vi "Double FFT Mesurament (Max Bin detection & CLK trick) test.vi"   [LabVIEW 2014]
uses:
  <vilib>/Platform/TimedLoop/XDataNode/timing_clust.ctl
  <vilib>/Platform/TimedLoop/XDataNode/nitl_modes.ctl
  <vilib>/Platform/TimedLoop/XDataNode/wakeup.ctl
  <vilib>/rvi/Analysis/measure/FFT/simModelSupport/niFPGA FFT Streaming Sim Properties.ctl
  <vilib>/rvi/Analysis/measure/FFT/simModelSupport/niFPGA FFT Sim Stream Group Properties.ctl
  <vilib>/rvi/Analysis/measure/FFT/simModelSupport/niFPGA FFT Sim Types.ctl
  <vilib>/rvi/Analysis/measure/FFT/simModelSupport/niFpgaFFTSimArithmeticProperties.ctl
  <vilib>/rvi/Analysis/measure/FFT/simModelSupport/niFpgaFFTSimDfxp.ctl
  <vilib>/fxp/LVFixedPointQuantizationPolicyTypeDef.ctl
  <vilib>/rvi/Analysis/measure/FFT/XNode/niFpgaFFTButterflyDelays.ctl
  <vilib>/rvi/Emulation/niFpgaSctlEmulationGetInTimedLoop.vi
  <vilib>/rvi/Emulation/niFpgaEmulationReportErrorSimple.vi
  <vilib>/rvi/Emulation/niFpgaGetClockAttributes.vi
  <vilib>/rvi/Emulation/niFpgaCriticalErrorInLSC.vi
  <vilib>/rvi/eio/common/nirviEmuTemplateMethod_errors.vi
  <vilib>/rvi/Emulation/niFpgaEmulationIsFPGAContextNoSignature.vi
  <vilib>/rvi/errors/niFpgaSetErrorForExecOnDevCompSimple.vi
  <vilib>/rvi/eio/common/nirviEmuReportErrorAndStop.vi
  <vilib>/rvi/DataTransferAndStorage/Container/Common/niFpgaContainerGetUniqueNameForEmu.vi
  <vilib>/rvi/FIFO/Fifo_Resource/nirvififoEmulationSetSize.vi
  <vilib>/rvi/FIFO/Fifo_Resource/nirviFifoEmulationQueueMgr.vi
  <instcachedir>/0/nirviFifoEmulationQueueMgr_E5CAEC123FF24DC58D834DCA3CDAA9B5.lvgen/nirviFifoEmulationQueueMgr_E5CAEC123FF24DC58D834DCA3CDAA9B5_005.vi
  <vilib>/Utility/error.llb/Clear Errors.vi
  <vilib>/rvi/FIFO/Fifo_Resource/nirvififoEmulationCreateLock.vi
  <vilib>/rvi/Emulation/niFpgaProcessEmulError.vi
  <vilib>/rvi/FIFO/Fifo_Resource/nirvififoEmulationObtainLock.vi
  <vilib>/rvi/FIFO/Fifo_Resource/nirvififoEmulationReleaseLock.vi
  <vilib>/rvi/occurrence/nirviWaitOnOccurrenceBase.vi
  <vilib>/rvi/errors/nirviReportUnexpectedCaseInternalError.vi
  <vilib>/rvi/errors/nirviReportUnexpectedCaseInternalError (U32).vi
  <vilib>/rvi/Memory/Memory_Emulation/niFpgaMemoryEmulationCacheClearOnFirstRun.vi
  <vilib>/rvi/Memory/Memory_Emulation/nirvimemoryEmulationManagerCache_MakeExclusive.vi
  <vilib>/rvi/Memory/Memory_Emulation/niFpgaMemoryEmulationValidateCache.vi
  <vilib>/rvi/Memory/Memory_Emulation/nirvimemoryEmulationManagerCache_InsertValue.vi
  <vilib>/rvi/Memory/Memory_Emulation/nirvimemoryEmulationManagerCache_ReleaseExclusive.vi
  <vilib>/rvi/Memory/Memory_Emulation/nirvimemoryEmulationManagerCache_GetValue.vi
  <vilib>/rvi/Memory/Memory_Emulation/nirvimemoryEmulationManagerCache_SetValue.vi
  <instcachedir>/0/nirviFifoEmulationQueueMgr_E5CAEC123FF24DC58D834DCA3CDAA9B5.lvgen/nirviFifoEmulationQueueMgr_E5CAEC123FF24DC58D834DCA3CDAA9B5_004.vi
  <vilib>/rvi/FIFO/Fifo_Resource/nirvififoEmulationDetermineInputValidOut.vi
  <vilib>/rvi/Memory/Memory_Emulation/nirvimemoryFastEmulation.vi
  <vilib>/rvi/Memory/Memory_Emulation/nirvimemoryEmulation.vi
  <vilib>/rvi/Analysis/measure/FFT/simModelSupport/niFpgaFFTSimModelStreamingCore.vi
  <vilib>/Platform/TimedLoop/XDataNode/XDataNode.xnode
  <vilib>/eio/EIOMethodNode/EIOMethodNode.xnode
  <vilib>/rvi/DataTransferAndStorage/Container/XNode/niFpgaContainer.xnode
  <vilib>/rvi/FIFO/Fifo_Resource/nirvififoEmulationRead.vi
  <vilib>/rvi/DataTransferAndStorage/Register/Emulation/niFpgaRegisterEmulation.vi
  <vilib>/rvi/FIFO/Fifo_Resource/nirvififoEmulationWrite.vi
  <vilib>/rvi/FIFO/Fifo_Resource/nirvififoEmulationGetNumberOfElementsToWrite.vi
  <vilib>/rvi/Analysis/measure/FFT/XNode/niFpgaFFT.xnode
  <vilib>/Platform/TimedLoop/XDataNode/XDNodeRunTimeDep.lvlib
types:
  T1 = typedef "XDNodeRunTimeDep.lvlib/timing_clust.ctl" = cluster{"Expected End [f-1]":u64, "Actual End [f-1]":u64, "Finished Late? [f-1]":bool, "Expected End [i-1]":u64, "Actual End [i-1]":u64, "Finished Late? [i-1]":bool, "Expected Start [i]":u64, "Actual Start [i]":u64, "Expected Start [f]":u64, "Actual Start [f]":u64, "Source Name":string, "Structure Name":string, "Period":i64, "Deadline":i64, "Offset":i64, "Start":i64, "Priority":i32, "Timeout":i32, "Mode":T2, "Wakeup Reason":T3, "Error":errorcluster, "Source Type":string, "Secondary Source Type":string, "Global End Time":u64, "Global Start Time":u64, "Frame Duration":u64, "Iteration Duration":u64, "Assigned CPU":i32, "I/O Scan Engine Mode":u32}
  T2 = typedef "XDNodeRunTimeDep.lvlib/nitl_modes.ctl" = enum32{"No Change", "Process missed periods, maintain original phase", "Discard missed periods, maintain original phase", "Process missed periods, ignore original phase", "Discard missed periods, ignore original phase"}
  T3 = typedef "XDNodeRunTimeDep.lvlib/wakeup.ctl" = enum32{"Normal", "Aborted", "Asynchronous wakeup", "Timing source error", "Timed loop error", "Timeout"}
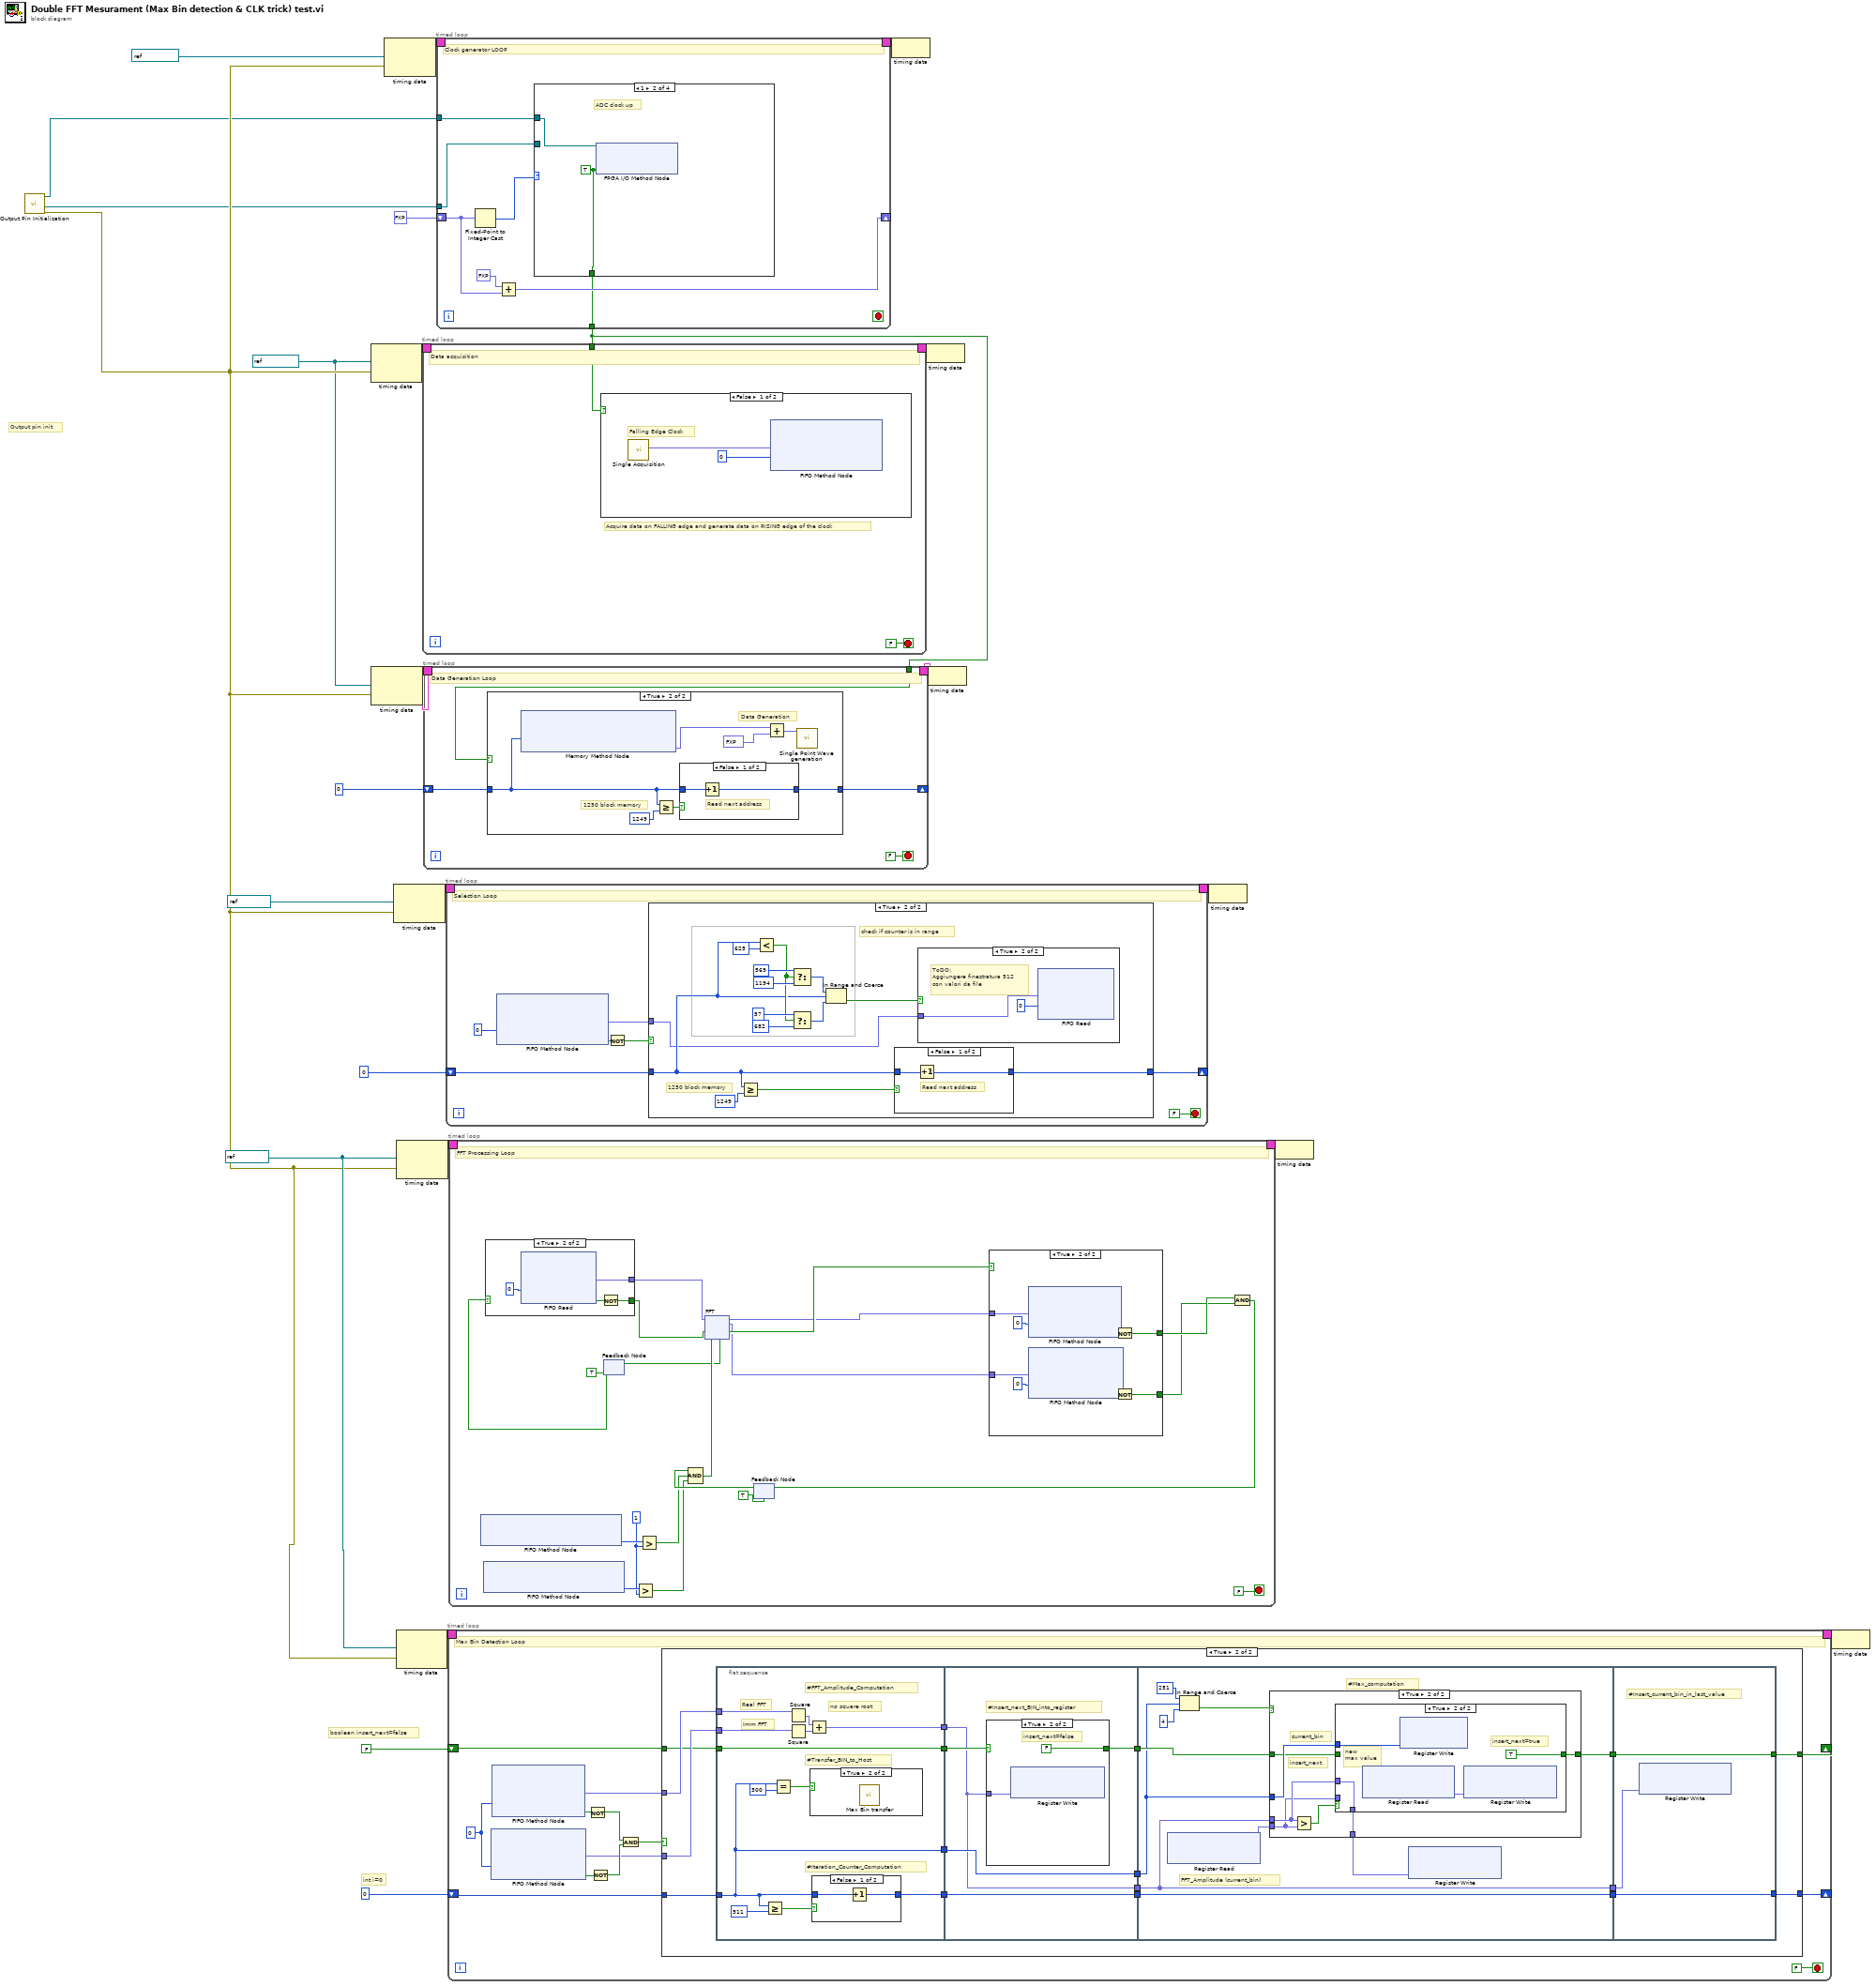
[diagram p0: block diagram]
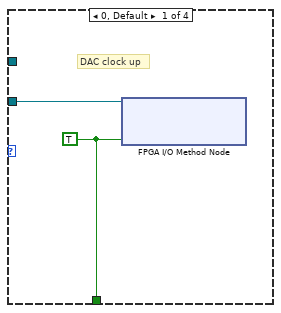
[diagram p2: hidden frame]
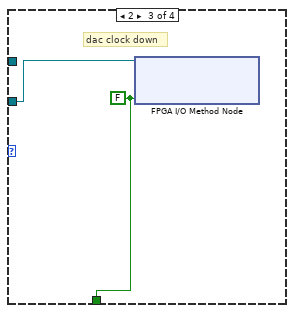
[diagram p3: hidden frame]
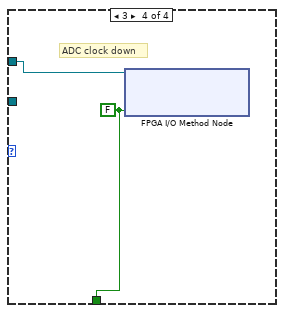
[diagram p4: hidden frame]
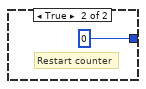
[diagram p7: hidden frame]
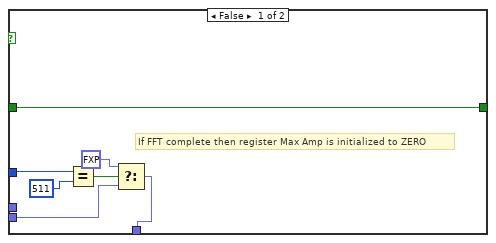
[diagram p9: hidden frame]
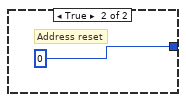
[diagram p13: hidden frame]
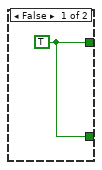
[diagram p14: hidden frame]
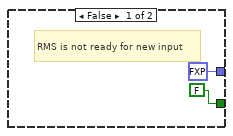
[diagram p15: hidden frame]
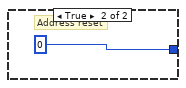
[diagram p17: hidden frame]
diagram:
  w11 = refnum<k21> "50MHz" ("Source Name")
  w2 = refnum<k21> "100MHz" ("Source Name")
  # "int i=0"
  # "boolean insert_next=false"
  # "Output pin init"
  n1 = call "Output Pin Initialization.vi"() -> ("error out"=w7:errorcluster, "I/O Out Clock DAC (pin16)"=w5:refnum<k21>, "I/O Out Clock ADC (pin17)"=w4:refnum<k21>)  [unwired: 8 in]
  n2 = node-c288(w2, w7) -> (w25:T1)
  n3 = node-c288(w2, w7) -> (w23:T1)
  n4 = node-c288(refnum<k21> "200MHz" ("Source Name"), w7) -> (w10:T1)
  n5 = node-c288(refnum<k21> "50MHz" ("Source Name"), w7) -> (w19:T1)
  n6 = node-c288(w11, w7) -> (w13:T1)
  n7 = node-c288(w11, w7) -> (w21:T1)
  n8 = timed-loop {
    timing: w10 -> [_]
    timing-out: [_] -> w9
    shift-right: [w29] -> _
    shift-left: fxp<+,2,2> 0.0 -> [w31]
    tunnel: w5 -> [w28]
    tunnel: [w27] -> w3
    tunnel: w4 -> [w26]
    stop <- _ stop-if-true
    # "Clock generator LOOP"
    n9 = Fixed-Point to Integer Cast(1:w31) -> (0:w32:u8)
    n10 = Add(x=fxp<+,2,2> 1.0, y=w31) -> (x+y=w29:fxp<+,2,2>)
    n11 = case shown="1" w32 {
      tunnel: w28 -> [w34 _ w38 _]
      tunnel: [w33 w35 w37 w39] -> w27
      tunnel: w26 -> [_ w36 _ w40]
      frame 0, Default {
        w33 = TRUE ("Data")
        # "DAC clock up"
        n12 = xnode "FPGA I/O Method Node"("FPGA I/O In"=w34, "Data"=w33) -> ()  [unwired: 1 out]
      }
      frame 1 {
        w35 = TRUE ("Data")
        # "ADC clock up"
        n13 = xnode "FPGA I/O Method Node"("FPGA I/O In"=w36, "Data"=w35) -> ()  [unwired: 1 out]
      }
      frame 2 {
        w37 = FALSE ("Data")
        # "dac clock down"
        n14 = xnode "FPGA I/O Method Node"("FPGA I/O In"=w38, "Data"=w37) -> ()  [unwired: 1 out]
      }
      frame 3 {
        w39 = FALSE ("Data")
        # "ADC clock down"
        n15 = xnode "FPGA I/O Method Node"("FPGA I/O In"=w40, "Data"=w39) -> ()  [unwired: 1 out]
      }
    }
  }
  n16 = timed-loop {
    timing: w25 -> [_]
    timing-out: [_] -> w24
    tunnel: w3 -> [w43]
    stop <- FALSE stop-if-true
    # "Acquire data on FALLING edge and generate data on RISING edge of the clock"
    # "Data acquisition"
    n17 = case shown="False" w43 {
      frame False {
        # "Falling Edge Clock"
        n18 = call "Single Acquisition.vi"() -> ("Out"=w46:fxp<+/-,12,12>)  [unwired: 10 in, 1 out]
        n19 = xnode ("FIFO Method Node")("Element"=w46, "Timeout"=0) -> ()  [unwired: 1 in, 2 out]
      }
      frame True {
      }
    }
  }
  n20 = timed-loop {
    timing: w23 -> [_]
    timing-out: [_] -> w22
    shift-right: [w52] -> _
    shift-left: u32 0 -> [w50]
    tunnel: w3 -> [w49]
    stop <- FALSE stop-if-true
    # "Data Generation Loop"
    n21 = case shown="True" w49 {
      tunnel: [w53 w58] -> w52
      tunnel: w50 -> [w53 w57]
      frame False {
      }
      frame True {
        # "Data Generation"
        # "1250 block memory"
        n22 = xnode ("Memory Method Node")("Address"=w57) -> ("Data"=w54:fxp<+/-,12,12>)  [unwired: 1 in, 1 out]
        n23 = Greater Or Equal?(x=w57, y=u32 1249) -> (x >= y?=w59:bool)
        n24 = case shown="False" w59 {
          tunnel: w57 -> [w62 _]
          tunnel: [w61 u32 0] -> w58
          frame False {
            # "Read next address"
            n25 = Increment(x=w62) -> (x+1=w61:u32)
          }
          frame True {
            # "Address reset"
          }
        }
        n26 = Add(x=w54, y=fxp<+,12,12> 2048.0) -> (x+y=w55:fxp<+/-,14,14>)
        n27 = call "Single Point Wave generation.vi"("Data To Write"=w55) -> ()  [unwired: 10 in, 1 out]
      }
    }
  }
  n28 = timed-loop {
    timing: w19 -> [_]
    timing-out: [_] -> w18
    shift-right: [w71] -> _
    shift-left: u32 0 -> [w70]
    stop <- FALSE stop-if-true
    # "Selection Loop"
    n29 = xnode ("FIFO Method Node")("Timeout"=0) -> ("Element"=w67:fxp<+/-,12,12>, "Timed Out?"=w68:bool)  [unwired: 1 in, 1 out]
    n30 = Not(x=w68) -> (.not. x?=w69:bool)
    n31 = case shown="True" w69 {
      tunnel: [w73 w85] -> w71
      tunnel: w70 -> [w73 w76]
      tunnel: w67 -> [_ w74]
      frame False {
      }
      frame True {
        # "check if counter is in range"
        # "1250 block memory"
        n32 = Greater Or Equal?(x=w76, y=u32 1249) -> (x >= y?=w86:bool)
        n33 = Less?(x=w76, y=u32 625) -> (x < y?=w77:bool)
        n34 = Select(t=u32 57 ("lower limit"), s=w77, f=u32 682 ("lower limit")) -> (s? t:f=w79:u32)
        n35 = Select(t=u32 569 ("upper limit"), s=w77, f=u32 1194 ("upper limit")) -> (s? t:f=w80:u32)
        n36 = In Range and Coerce(upper limit=w80, x=w76, lower limit=w79) -> (In Range?=w75:bool)  [unwired: 1 out]
        n37 = case shown="False" w86 {
          tunnel: w76 -> [w91 _]
          tunnel: [w90 u32 0] -> w85
          frame False {
            # "Read next address"
            n38 = Increment(x=w91) -> (x+1=w90:u32)
          }
          frame True {
            # "Address reset"
          }
        }
        n39 = case shown="True" w75 {
          tunnel: w74 -> [_ w89]
          frame False {
          }
          frame True {
            # "ToDO:\nAggiungere finestratura 512\ncon valori da file"
            n40 = xnode ("FIFO Read")("Element"=w89, "Timeout"=0) -> ()  [unwired: 1 in, 2 out]
          }
        }
      }
    }
  }
  n41 = timed-loop {
    shift-right: [w98] -> _
    shift-left: 0 ("Timeout") -> [w99]
    shift-right: [w96] -> _
    shift-left: FALSE -> [w97]
    timing: w13 -> [_]
    timing-out: [_] -> w12
    stop <- FALSE stop-if-true
    w107 = 0 ("Timeout")
    # "Max Bin Detection Loop"
    n42 = xnode ("FIFO Method Node")("Timeout"=w107) -> ("Element"=w100:fxp<+/-,22,22>, "Timed Out?"=w105:bool)  [unwired: 1 in, 1 out]
    n43 = xnode ("FIFO Method Node")("Timeout"=w107) -> ("Element"=w101:fxp<+/-,22,22>, "Timed Out?"=w106:bool)  [unwired: 1 in, 1 out]
    n44 = Not(x=w106) -> (.not. x?=w104:bool)
    n45 = Not(x=w105) -> (.not. x?=w103:bool)
    n46 = And(x=w104, y=w103) -> (x .and. y?=w102:bool)
    n47 = case shown="True" w102 {
      tunnel: w101 -> [_ w126]
      tunnel: w100 -> [_ w125]
      tunnel: w99 -> [w109 w123]
      tunnel: [w109 w110] -> w98
      tunnel: w97 -> [w108 w117]
      tunnel: [w108 w112] -> w96
      frame False {
        # "Data are NOT ready in Target Real FFT and Target Imm FFT FIFOs"
      }
      frame True {
        n48 = flat-sequence {
          tunnel: w126 -> [w135]
          tunnel: w125 -> [w136]
          tunnel: [w134] -> w124
          tunnel: w123 -> [w127]
          tunnel: [w133] -> w122
          tunnel: [w127] -> w119
          tunnel: [w130] -> w118
          tunnel: w117 -> [w130]
          tunnel: w124 -> [w143]
          tunnel: w122 -> [w146]
          tunnel: [w146] -> w121
          tunnel: w119 -> [w144]
          tunnel: w118 -> [w145]
          tunnel: [w144] -> w116
          tunnel: [w143] -> w115
          tunnel: [w142] -> w114
          tunnel: w121 -> [w159]
          tunnel: [w159] -> w120
          tunnel: w116 -> [w152]
          tunnel: w115 -> [w154]
          tunnel: w114 -> [w155]
          tunnel: [w154] -> w113
          tunnel: [w153] -> w111
          tunnel: w120 -> [w180]
          tunnel: w113 -> [w182]
          tunnel: w111 -> [w181]
          tunnel: [w181] -> w112
          tunnel: [w180] -> w110
          frame #0 {
            # "no square root"
            # "#Transfer_BIN_to_Host"
            # "#Iteration_Counter_Computation"
            # "#FFT_Amplitude_Computation"
            # "Imm FFT"
            # "Real FFT"
            n49 = Greater Or Equal?(x=w127, y=511) -> (x >= y?=w131:bool)
            n50 = Equal?(x=w127, y=300) -> (x = y?=w129:bool)
            n51 = Square(x=w135) -> (x^2=w138:fxp<+,43,43>)
            n52 = Square(x=w136) -> (x^2=w137:fxp<+,43,43>)
            n53 = Add(x=w138, y=w137) -> (x+y=w134:fxp<+,44,44>)
            n54 = case shown="True" w129 {
              frame False {
                # "FFT Comp is NOT finished"
              }
              frame True {
                n55 = call "Max Bin transfer.vi"() -> ()  [unwired: 11 in, 1 out]
              }
            }
            n56 = case shown="False" w131 {
              tunnel: w127 -> [w139 _]
              tunnel: [w140 0 ("Timeout")] -> w133
              frame False {
                n57 = Increment(x=w139) -> (x+1=w140:i32)
              }
              frame True {
                # "Restart counter"
              }
            }
          }
          frame #1 {
            # "#Insert_next_BIN_into_register"
            n58 = case shown="True" w145 {
              selector: w145 -> [w147 _]
              tunnel: [w147 FALSE] -> w142
              tunnel: w143 -> [_ w148]
              frame False {
              }
              frame True {
                # "insert_next=false"
                n59 = xnode ("Register Write")("Data"=w148) -> ()  [unwired: 1 in, 1 out]
              }
            }
          }
          frame #2 {
            # "FFT_Amplitude (current_bin)"
            # "#Max_computation"
            n60 = xnode ("Register Read")() -> ("Data"=w151:fxp<+,44,44>)  [unwired: 1 in, 1 out]
            n61 = In Range and Coerce(upper limit=251, x=w152, lower limit=4) -> (In Range?=w156:bool)  [unwired: 1 out]
            n62 = case shown="True" w156 {
              tunnel: w154 -> [_ w172]
              tunnel: w152 -> [w164 w171]
              tunnel: w155 -> [w166 w170]
              tunnel: [w166 w169] -> w153
              tunnel: w151 -> [w162 w167]
              tunnel: [w160 w168] -> w150
              frame False {
                # "If FFT complete then register Max Amp is initialized to ZERO"
                n63 = Equal?(x=w164, y=511) -> (x = y?=w165:bool)
                n64 = Select(t=fxp<+,44,44> 0.0, s=w165, f=w162) -> (s? t:f=w160:fxp<+,44,44>)
              }
              frame True {
                # "insert_next"
                # "current_bin"
                n65 = Greater?(x=w172, y=w167) -> (0:w173:bool)
                n66 = case shown="True" w173 {
                  tunnel: w172 -> [_ w176]
                  tunnel: w171 -> [_ w179]
                  tunnel: w170 -> [w175 _]
                  tunnel: [w175 TRUE] -> w169
                  tunnel: [w174 w176] -> w168
                  tunnel: w167 -> [w174 _]
                  frame False {
                    # "Old value is re-written"
                  }
                  frame True {
                    # "new\nmax value"
                    # "insert_next=true"
                    n67 = xnode ("Register Read")() -> ("Data"=w177:fxp<+,44,44>)  [unwired: 1 in, 1 out]
                    n68 = xnode ("Register Write")("Data"=w179) -> ()  [unwired: 1 in, 1 out]
                    n69 = xnode ("Register Write")("Data"=w177) -> ()  [unwired: 1 in, 1 out]
                  }
                }
              }
            }
            n70 = xnode ("Register Write")("Data"=w150) -> ()  [unwired: 1 in, 1 out]
          }
          frame #3 {
            # "#Insert_current_bin_in_last_value"
            n71 = xnode ("Register Write")("Data"=w182) -> ()  [unwired: 1 in, 1 out]
          }
        }
      }
    }
  }
  n72 = timed-loop {
    timing: w21 -> [_]
    timing-out: [_] -> w20
    stop <- FALSE stop-if-true
    w187 = u32 1 ("y")
    # "FFT Processing Loop"
    n73 = xnode ("FIFO Method Node")() -> ("Number of Elements to Write"=w189:u32)  [unwired: 1 in, 1 out]
    n74 = xnode ("FIFO Method Node")() -> ("Number of Elements to Write"=w188:u32)  [unwired: 1 in, 1 out]
    n75 = feedback #1(TRUE ("ready for input")) -> (w204:bool)
    n76 = case shown="True" w204 {
      tunnel: [FALSE w245] -> w198
      tunnel: [fxp<+/-,12,12> 0.0 ("Element") w242] -> w199
      frame False {
        # "RMS is not ready for new input"
      }
      frame True {
        n77 = xnode ("FIFO Read")("Timeout"=0) -> ("Element"=w242:fxp<+/-,12,12>, "Timed Out?"=w244:bool)  [unwired: 1 in, 1 out]
        n78 = Not(x=w244) -> (.not. x?=w245:bool)
      }
    }
    n79 = Greater?(x=w188, y=w187) -> (0:w185:bool)
    n80 = Greater?(x=w189, y=w187) -> (0:w186:bool)
    n81 = feedback #2(TRUE) -> (w200:bool)
    n82 = Compound Arithmetic op=AND(w200, w186, w185) -> (w197:bool)
    n83 = xnode "FFT"("real data in"=w199, "input valid"=w198, "ready for output"=w197) -> ("ready for input"=w196:bool, "real data out"=w194:fxp<+/-,22,22>, "imaginary data out"=w193:fxp<+/-,22,22>, "output valid"=w195:bool)  [unwired: 2 in, 1 out]
    n84 = feedback-in #1(w196) -> ()
    n85 = case shown="True" w195 {
      tunnel: w194 -> [_ w239]
      tunnel: w193 -> [_ w238]
      tunnel: [w231 w237] -> w192
      tunnel: [w231 w236] -> w191
      frame False {
        w231 = TRUE
      }
      frame True {
        n86 = xnode ("FIFO Method Node")("Element"=w239, "Timeout"=0) -> ("Timed Out?"=w232:bool)  [unwired: 1 in, 1 out]
        n87 = xnode ("FIFO Method Node")("Element"=w238, "Timeout"=0) -> ("Timed Out?"=w233:bool)  [unwired: 1 in, 1 out]
        n88 = Not(x=w232) -> (.not. x?=w237:bool)
        n89 = Not(x=w233) -> (.not. x?=w236:bool)
      }
    }
    n90 = Compound Arithmetic op=AND(w192, w191) -> (w190:bool)
    n91 = feedback-in #2(w190) -> ()
  }
  n92 = node-c288(w9) -> ()
  n93 = node-c288(w24) -> ()
  n94 = node-c288(w22) -> ()
  n95 = node-c288(w18) -> ()
  n96 = node-c288(w20) -> ()
  n97 = node-c288(w12) -> ()
